vi "Disconnect from Library.vi"(8 "error in (no error)":errorcluster, 11 "Mock Class Path":path=path "C:/Users/AntonSundqvist/Desktop/New folder/test.lvclass") -> (0 "error out":errorcluster, 2 "Owner":refnum<vi>, 3 "Mock Class Path Out":path=path "C:/Users/AntonSundqvist/Desktop/New folder/test.lvclass")   [LabVIEW 2020, in "Mock Class Updater.lvclass"]
uses:
  Mock Class Updater.lvclass
  Mock Class Updater.lvclass/Mock Class Updater.ctl
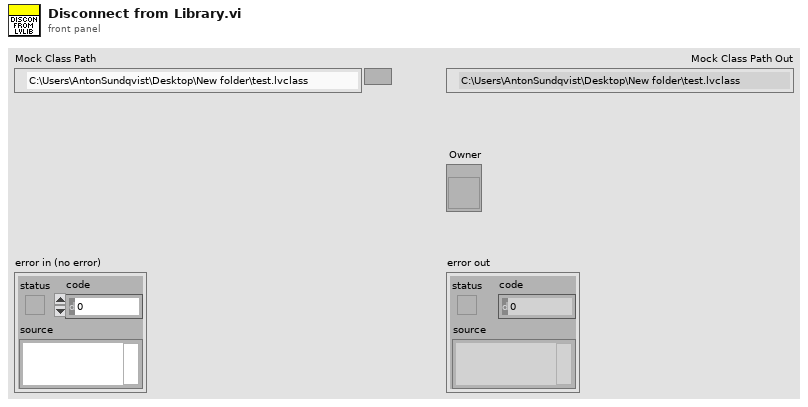
[diagram p1: front panel]
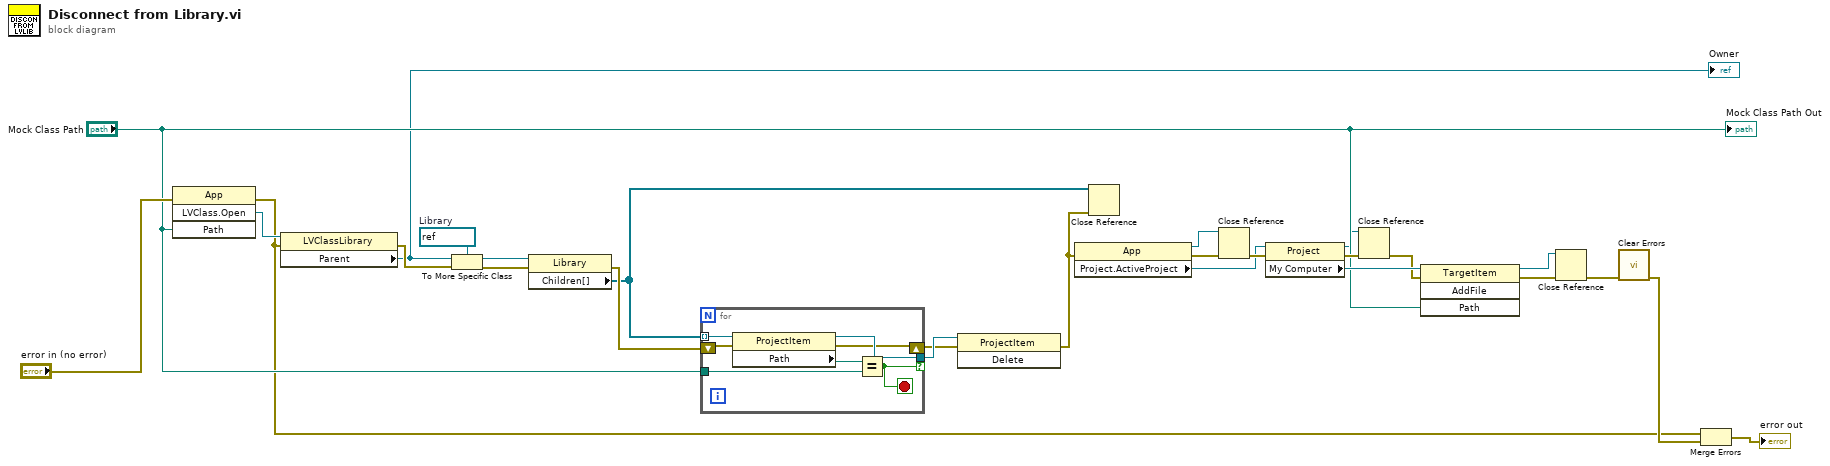
[diagram p0: block diagram]
diagram:
  w26 = refnum<vi> refnum  # Library
  n1 = invoke class="App" method="LVClass.Open"(error in="error in (no error)", "Path"="Mock Class Path") -> (error out=w2:errorcluster, "LVClass.Open"=w27:refnum<vi>)  [unwired: 2 in, 2 out]
  n2 = property class="LVClassLibrary"(reference=w27, error in=w2) -> (error out=w3:errorcluster, "Parent"=w1:refnum<vi>)  [unwired: 1 out]
  "Owner" <- w1
  n3 = To More Specific Class(target class=w26, reference=w1, error in=w3) -> (specific class reference=w25:refnum<vi>, error out=w24:errorcluster)
  n4 = property class="Library"(reference=w25, error in=w24) -> (error out=w21:errorcluster, "Children[]"=w10:refnum<vi>[])  [unwired: 1 out]
  n5 = for {
    tunnel: w10 -> [w34] mode=indexing
    tunnel: [w32] -> w23 if=w30
    tunnel: "Mock Class Path" -> [w31]
    shift-right: [w28] -> w22
    shift-left: w21 -> [w29]
    stop <- w30 stop-if-true
    n6 = property class="ProjectItem"(reference=w34, error in=w29) -> (reference out=w32:refnum<vi>, error out=w28:errorcluster, "Path"=w33:path)
    n7 = Equal?(x=w33, y=w31) -> (x = y?=w30:bool)
  }
  n8 = invoke class="ProjectItem" method="Delete"(reference=w23, error in=w22) -> (error out=w11:errorcluster)  [unwired: 1 in, 2 out]
  n9 = property class="App"(error in=w11) -> (reference out=w19:refnum<vi>, error out=w17:errorcluster, "Project.ActiveProject"=w16:refnum<vi>)  [unwired: 1 in]
  n10 = Close Reference(reference=w10, error in (no error)=w11) -> ()  [unwired: 1 out]
  n11 = Close Reference(reference=w19, error in (no error)=w17) -> (error out=w18:errorcluster)
  n12 = property class="Project"(reference=w16, error in=w18) -> (reference out=w8:refnum<vi>, error out=w14:errorcluster, "My Computer"=w15:refnum<vi>)
  n13 = Close Reference(reference=w8, error in (no error)=w14) -> (error out=w9:errorcluster)
  n14 = invoke class="TargetItem" method="AddFile"(reference=w15, error in=w9, "Path"="Mock Class Path") -> (reference out=w6:refnum<vi>, error out=w13:errorcluster)  [unwired: 1 in, 2 out]
  n15 = Close Reference(reference=w6, error in (no error)=w13) -> (error out=w7:errorcluster)
  n16 = call <vilib>:"Clear Errors.vi"("error in (no error)"=w7) -> ("error out"=w5:errorcluster)  [unwired: 5 in, 1 out]
  n17 = Merge Errors(w2, w5) -> (→"error out":errorcluster)
  "Mock Class Path Out" <- "Mock Class Path"
